vi "Write params.vi"(8 "error in (no error)":errorcluster, 10 "output":T1, 11 "Simulated Oscilloscope in":refnum<class "Simulated Oscilloscope.lvclass">) -> (0 "error out":errorcluster, 3 "Simulated Oscilloscope out":refnum<class "Simulated Oscilloscope.lvclass">)   [LabVIEW 2014, in "Simulated Oscilloscope.lvclass"]
uses:
  Simulated Oscilloscope.lvclass
  Params.ctl
  Simulated Oscilloscope.lvclass/Simulated Oscilloscope.ctl
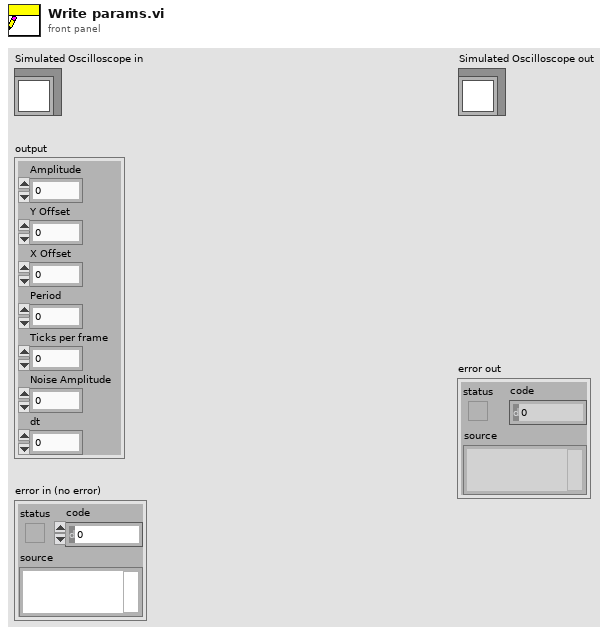
[diagram p1: front panel]
types:
  T1 = typedef "Simulated Oscilloscope.lvclass/Params.ctl" = cluster{"Amplitude":dbl, "Y Offset":dbl, "X Offset":dbl, "Period":dbl, "Ticks per frame":dbl, "Noise Amplitude":dbl, "dt":dbl}
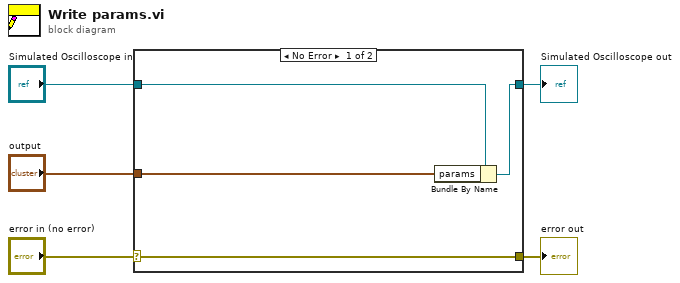
[diagram p0: block diagram]
diagram:
  n1 = case shown="No Error" "error in (no error)" {
    selector: "error in (no error)" -> [w9 w10]
    tunnel: [w9 w10] -> w4
    tunnel: [w7 w11] -> w2
    tunnel: "Simulated Oscilloscope in" -> [w8 w11]
    tunnel: "output" -> [w6 _]
    frame No Error {
      n2 = Bundle By Name(cluster=w8, "params"=w6) -> (w7:refnum<class "Simulated Oscilloscope.lvclass">)
    }
    frame Error {
    }
  }
  "error out" <- w4
  "Simulated Oscilloscope out" <- w2
